vi "Write Fast FPGA Telem to FIFO.vi"   [LabVIEW 2015]
uses:
  FPGA Telem for Fast Logging.ctl
  <vilib>/FPGAPlugInAG/Dynamic/niLvFpga_Close_Dynamic.vi
  <vilib>/rvi/errors/niLvFpgaAdjustHostInterfaceError.vi
  <vilib>/Utility/error.llb/Error Cluster From Error Code.vi
  Global Data.vi
  <vilib>/rvi/interface/common/dynamic/niFpgaDynamicAddResources.vi
  <vilib>/FPGAPlugInAG/sbRIO-9627/niLvFpga_Open_sbRIO-9627.vi
  <vilib>/rvi/interface/nirviCloseFPGA/nirviCloseFPGA.xnode
  <vilib>/rvi/interface/nirviReadWriteControl/nirviReadWriteControl.xnode
  <vilib>/rvi/interface/nirviOpenFPGA/nirviOpenFPGA.xnode
  FPGA Bitfiles/Latest.lvbitx
  NiFpgaLv.dll
  <vilib>/rvi/interface/Simulation/niFpgaSimulationCallBeginRW.vi
types:
  T1 = typedef "FPGA Telem for Fast Logging.ctl" = cluster{"Time Stamp":timestamp, "tRequestMCControl":dbl, "rAverageThrottle":dbl, "rTPS2":fxp<+/-,31,22>, "rTPS1":fxp<+/-,31,22>, "rThrottle":fxp<+/-,33,22>, "aSteerWheel":fxp<+/-,31,13>, "pBrakeR":fxp<+,26,13>, "pBrakeF":fxp<+,26,13>, "ILowCurrent":fxp<+/-,24,15>, "IHighCurrent":fxp<+/-,24,15>, "nWheelFL":fxp<+/-,32,16>, "nWheelFR":fxp<+/-,32,16>, "nWheelRL":fxp<+/-,32,16>, "nWheelRR":fxp<+/-,32,16>, "gXiPhone":dbl, "gYiPhone":dbl, "gZiPhone":dbl, "nYawXiPhone":dbl, "nYawYiPhone":dbl, "nYawZiPhone":dbl, "vWheelRR":fxp<+/-,32,18>, "vWheelRL":fxp<+/-,32,18>, "vWheelFR":fxp<+/-,32,18>, "vWheelFL":fxp<+/-,32,18>, "vWheelLowest":fxp<+/-,32,18>, "vWheelHighest":fxp<+/-,32,18>, "vAxleF":fxp<+/-,33,19>, "vCar":fxp<+/-,33,19>, "sLap":fxp<+,32,12>, "rSlipRL":fxp<+/-,12,1>, "rSlipRR":fxp<+/-,12,1>, "rSlipFL":fxp<+/-,12,1>, "rSlipFR":fxp<+/-,12,1>, "MPowerLimiterCorrection":dbl}
  T2 = cluster{"read mode":enum16{"polling", "blocking"}, "write mode":enum16{"polling", "blocking"}}
  T3 = cluster{"Accel X":dbl, "Accel Y":dbl, "Accel Z":dbl, "Gyro X":dbl, "Gyro Y":dbl, "Gyro Z":dbl}
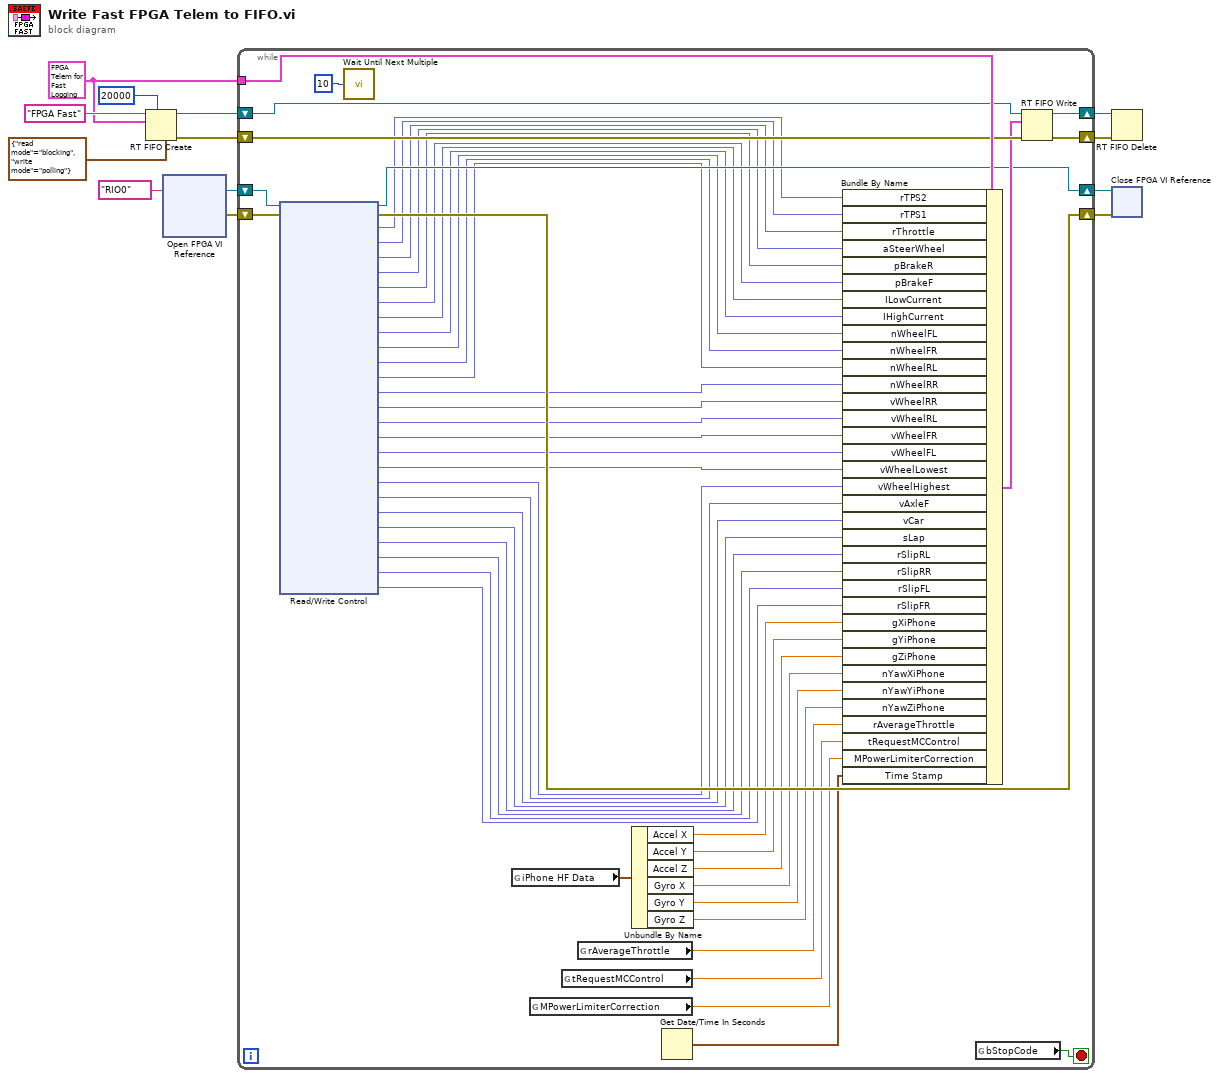
[diagram p0: block diagram]
diagram:
  w2 = T1 {"Time Stamp"=timestamp(0 s since 1904-01-01), "tRequestMCControl"=0.0, "rAverageThrottle"=0.0, "rTPS2"=0.421875, "rTPS1"=0.69921875, "rThrottle"=0.0, "aSteerWheel"=0.0078125, "pBrakeR"=186.34033203125, "pBrakeF"=185.44775390625, "ILowCurrent"=0.48046875, "IHighCurrent"=0.482421875, "nWheelFL"=0.0, "nWheelFR"=0.0, "nWheelRL"=0.0, "nWheelRR"=0.0, "gXiPhone"=0.0, "gYiPhone"=0.0, "gZiPhone"=0.0, "nYawXiPhone"=0.0, "nYawYiPhone"=0.0, "nYawZiPhone"=0.0, "vWheelRR"=0.0, "vWheelRL"=0.0, "vWheelFR"=0.0, "vWheelFL"=0.0, "vWheelLowest"=0.0, "vWheelHighest"=0.0, "vAxleF"=0.0, "vCar"=0.0, "sLap"=0.0, "rSlipRL"=0.0, "rSlipRR"=0.0, "rSlipFL"=0.0, "rSlipFR"=0.0, "MPowerLimiterCorrection"=0.0} ("FPGA Fast Telem")
  n1 = RT FIFO Create(0:"FPGA Fast" ("name (unnamed)"), 1:w2, 4:u32 20000 ("size (10)"), 7:T2 {"read mode"=enum."blocking", "write mode"=enum."polling"} ("r/w modes (polling,polling)")) -> (8:w8:refnum<k33>, 11:w7:errorcluster)  [unwired: 4 in, 1 out]
  n2 = xnode "Open FPGA VI Reference"("resource name"=tag "RIO0") -> ("FPGA VI Reference Out"=w13:refnum<k20>, "error out"=w12:errorcluster)  [unwired: 1 in]
  n3 = while {
    tunnel: w2 -> [w61]
    shift-right: [w55] -> w5
    shift-left: w8 -> [w58]
    shift-right: [w54] -> w6
    shift-left: w7 -> [w57]
    shift-right: [w53] -> w4
    shift-left: w13 -> [w60]
    shift-right: [w52] -> w3
    shift-left: w12 -> [w59]
    stop <- w37 stop-if-true
    n4 = xnode "Read/Write Control"("FPGA VI Reference In"=w60, "error in"=w59) -> ("FPGA VI Reference Out"=w53:refnum<k20>, "error out"=w52:errorcluster, "rTPS2"=w49:fxp<+/-,31,22>, "rTPS1"=w48:fxp<+/-,31,22>, "rThrottle"=w47:fxp<+/-,33,22>, "aSteerWheel"=w46:fxp<+/-,22,10>, "pBrakeR"=w45:fxp<+,26,13>, "pBrakeF"=w44:fxp<+,26,13>, "ILowCurrent"=w43:fxp<+/-,19,15>, "IHighCurrent"=w42:fxp<+/-,19,15>, "nWheelFL"=w41:fxp<+/-,29,16>, "nWheelFR"=w40:fxp<+/-,29,16>, "nWheelRL"=w39:fxp<+/-,29,16>, "nWheelRR"=w38:fxp<+/-,29,16>, "vWheelRR"=w36:fxp<+/-,32,18>, "vWheelRL"=w35:fxp<+/-,32,18>, "vWheelFR"=w34:fxp<+/-,32,18>, "vWheelFL"=w33:fxp<+/-,32,18>, "vWheelLowest"=w32:fxp<+/-,32,18>, "vWheelHighest"=w31:fxp<+/-,32,18>, "vAxleF"=w30:fxp<+/-,33,19>, "vCar"=w29:fxp<+/-,33,19>, "sLap"=w28:fxp<+,32,12>, "rSlipRL"=w27:fxp<+/-,12,1>, "rSlipRR"=w26:fxp<+/-,12,1>, "rSlipFL"=w25:fxp<+/-,12,1>, "rSlipFR"=w24:fxp<+/-,12,1>)
    n5 = call "Wait Until Next Multiple"("Count(mSec)"=u32 10) -> ()  [unwired: 1 out]
    n6 = global read "Global Data.vi" "iPhone HF Data"() -> (w51:T3)
    n7 = global read "Global Data.vi" "MPowerLimiterCorrection"() -> (w14:dbl)
    n8 = global read "Global Data.vi" "tRequestMCControl"() -> (w22:dbl)
    n9 = global read "Global Data.vi" "rAverageThrottle"() -> (w21:dbl)
    n10 = Unbundle By Name(w51) -> ("Accel X"=w20:dbl, "Accel Y"=w19:dbl, "Accel Z"=w18:dbl, "Gyro X"=w17:dbl, "Gyro Y"=w16:dbl, "Gyro Z"=w15:dbl)
    n11 = Get Date/Time In Seconds() -> (seconds since 1Jan1904=w23:timestamp)
    n12 = Bundle By Name(cluster=w61, "rTPS2"=w49, "rTPS1"=w48, "rThrottle"=w47, "aSteerWheel"=w46, "pBrakeR"=w45, "pBrakeF"=w44, "ILowCurrent"=w43, "IHighCurrent"=w42, "nWheelFL"=w41, "nWheelFR"=w40, "nWheelRL"=w39, "nWheelRR"=w38, "vWheelRR"=w36, "vWheelRL"=w35, "vWheelFR"=w34, "vWheelFL"=w33, "vWheelLowest"=w32, "vWheelHighest"=w31, "vAxleF"=w30, "vCar"=w29, "sLap"=w28, "rSlipRL"=w27, "rSlipRR"=w26, "rSlipFL"=w25, "rSlipFR"=w24, "gXiPhone"=w20, "gYiPhone"=w19, "gZiPhone"=w18, "nYawXiPhone"=w17, "nYawYiPhone"=w16, "nYawZiPhone"=w15, "rAverageThrottle"=w21, "tRequestMCControl"=w22, "MPowerLimiterCorrection"=w14, "Time Stamp"=w23) -> (w56:T1)
    n13 = global read "Global Data.vi" "bStopCode"() -> (w37:bool)
    n14 = RT FIFO Write(0:w58, 1:w56, 3:w57) -> (8:w55:refnum<k33>, 11:w54:errorcluster)  [unwired: 2 in, 2 out]
  }
  n15 = RT FIFO Delete(0:w5, 3:w6) -> ()  [unwired: 1 in, 1 out]
  n16 = xnode "Close FPGA VI Reference"("FPGA VI Reference In"=w4, "error in"=w3) -> ()  [unwired: 1 out]
